vi "ProvaRobot.vi"() -> ()   [LabVIEW 2017]
uses:
  Sub VIs/Utilities/Start Boolean.ctl
  <vilib>/Platform/TimedLoop/XDataNode/timing_clust.ctl
  <vilib>/Platform/TimedLoop/XDataNode/nitl_modes.ctl
  <vilib>/Platform/TimedLoop/XDataNode/wakeup.ctl
  <vilib>/rvi/eio/common/nirviEmuTemplateMethod_errors.vi
  <vilib>/rvi/Emulation/niFpgaCriticalErrorInLSC.vi
  <vilib>/rvi/Emulation/niFpgaGetClockAttributes.vi
  <vilib>/rvi/Emulation/niFpgaEmulationReportErrorSimple.vi
  <vilib>/rvi/Emulation/niFpgaSctlEmulationGetInTimedLoop.vi
  <vilib>/rvi/eio/common/nirviEmuReportErrorAndStop.vi
  <vilib>/rvi/DataTransferAndStorage/Container/Common/niFpgaContainerSetEmuInfo.vi
  <vilib>/rvi/DataTransferAndStorage/Container/Common/niFpgaContainerGetUniqueNameForEmu.vi
  <vilib>/rvi/Emulation/niFpgaProcessEmulError.vi
  <vilib>/rvi/FIFO/Fifo_Resource/nirvififoEmulationDetermineInputValidOut.vi
  <vilib>/rvi/errors/nirviReportUnexpectedCaseInternalError.vi
  <vilib>/rvi/errors/nirviReportUnexpectedCaseInternalError (U32).vi
  <vilib>/rvi/occurrence/nirviWaitOnOccurrenceBase.vi
  <vilib>/rvi/FIFO/Fifo_Resource/nirvififoEmulationReleaseLock.vi
  <vilib>/rvi/FIFO/Fifo_Resource/nirvififoEmulationObtainLock.vi
  <vilib>/rvi/FIFO/Fifo_Resource/nirvififoEmulationCreateLock.vi
  <vilib>/rvi/FIFO/Fifo_Resource/nirvififoEmulationSetSize.vi
  <vilib>/rvi/FIFO/Fifo_Resource/nirviFifoEmulationQueueMgr.vi
  <instcachedir>/0/nirviFifoEmulationQueueMgr_E5CAEC123FF24DC58D834DCA3CDAA9B5.lvgen/nirviFifoEmulationQueueMgr_E5CAEC123FF24DC58D834DCA3CDAA9B5_000.vi
  <vilib>/rvi/errors/niFpgaSetErrorForExecOnDevCompSimple.vi
  <vilib>/rvi/Emulation/niFpgaEmulationIsFPGAContextNoSignature.vi
  <vilib>/Utility/error.llb/Clear Errors.vi
  <vilib>/Platform/TimedLoop/XDataNode/XDataNode.xnode
  <vilib>/eio/EIOMethodNode/EIOMethodNode.xnode
  <vilib>/eio/EIONode/EIONode.xnode
  <vilib>/rvi/LocalResourceManager/LocalResourceManager.xnode
  <vilib>/rvi/DataTransferAndStorage/Container/XNode/niFpgaContainer.xnode
  <vilib>/rvi/FIFO/Fifo_Resource/nirvififoEmulationWrite.vi
  <vilib>/rvi/FIFO/Fifo_Resource/nirvififoEmulationRead.vi
  <vilib>/Platform/TimedLoop/XDataNode/XDNodeRunTimeDep.lvlib
panel:
  in  "enable aux":bool
  in  "Numeric":u8
  in  "invertiM4":bool=TRUE
  in  "InvertiM3":bool=TRUE
  in  "InvertiM2":bool=TRUE
  in  "InvertiM1":bool=TRUE
  in  "DIO.C_0:7_write 2":u8 format="%08b"
  in  "ENB_AB 2":bool
  in  "ENB_AB":bool
  in  "DO.LED3:0":u8 format="%04b"
  out "DI.BTN":u8 format="%08b"
  in  "IRQ.DI_BTN.ENA":bool
  in  "IRQ.DI_BTN.RISE":bool
  in  "IRQ.DI_BTN.FALL":bool
  in  "IRQ.DI_BTN.CNT":u32
  in  "IRQ.DI_BTN.NO":u8
  out "AI.A_0.VAL":u16
  out "AI.A_1.VAL":u16
  out "AI.A_2.VAL":u16
  out "AI.A_3.VAL":u16
  out "AI.B_0.VAL":u16
  out "AI.B_1.VAL":u16
  out "AI.B_2.VAL":u16
  out "AI.B_3.VAL":u16
  out "AI.AudioIn_L.VAL":u16
  out "AI.AudioIn_R.VAL":u16
  out "AI.C_1.VAL":u16
  out "AI.C_0.VAL":u16
  in  "IRQ.AI_A_3:0.CNFG":u8 format="%.0b"
  in  "IRQ.AI_A_0.THRESHOLD":u16
  in  "IRQ.AI_A_1.THRESHOLD":u16
  in  "IRQ.AI_A_0.NO":u8
  in  "IRQ.AI_A_1.NO":u8
  in  "IRQ.AI_A_1.HYSTERESIS":u16=17
  in  "IRQ.AI_A_0.HYSTERESIS":u16=17
  in  "IRQ.TIMER.SETTIME":T1
  in  "IRQ.TIMER.WRITE":u32
  out "IRQ.TIMER.READ":u32
  out "SYS.RDY":bool
  out "SYS.AI.RDY":bool
  out "ACC.Z.VAL":u16
  out "SYS.ACC.RDY":bool
  out "ACC.Y.VAL":u16
  out "ACC.X.VAL":u16
  in  "StartShiftReg":bool
  in  "enable cannon":bool
  in  "SYS.SELECTA":u8 format="%08b"
  in  "DIO.A_15:8.OUT":u8 format="%08b"
  in  "DIO.A_15:8.DIR":u8 format="%08b"
  in  "I2C.A.DATO":u8
  out "I2C.A.DATI":u8
  in  "I2C.A.ADDR":u8 format="%08b"
  in  "I2C.A.CNTR":u8=213
  in  "I2C.A.CNTL":u8 format="%08b"
  out "I2C.A.STAT":u8 format="%08b"
  in  "I2C.A.CNFG":u8=1 format="%08b"
  in  "I2C.A.GO":T1
  in  "PWM period motor 4":u16=4000
  in  "Duty cycle motor 4":i16
  in  "PWM period motor 3":u16=4000
  in  "Duty cycle motor 3":i16
  out "deltaT motor 4":i32
  in  "Clear Overflow? 7":bool
  out "StatusEnc 7":u8
  out "Count encoder motor 4":u32
  in  "Reset encoder motor 4":bool
  out "deltaT motor 3":i32
  in  "Clear Overflow? 6":bool
  out "StatusEnc 6":u8
  out "Count encoder motor 3":u32
  in  "Reset encoder motor 3":bool
  in  "Reset encoder motor 1":bool
  out "Count encoder motor 1":u32
  out "StatusEnc 5":u8
  in  "Clear Overflow? 5":bool
  out "deltaT motor 1":i32
  in  "Reset encoder motor 2":bool
  out "Count encoder motor 2":u32
  out "StatusEnc 4":u8
  in  "Clear Overflow? 4":bool
  out "deltaT motor 2":i32
  in  "Duty cycle motor 1":i16
  in  "PWM period motor 1":u16=4000
  in  "Duty cycle motor 2":i16
  in  "PWM period motor 2":u16=4000
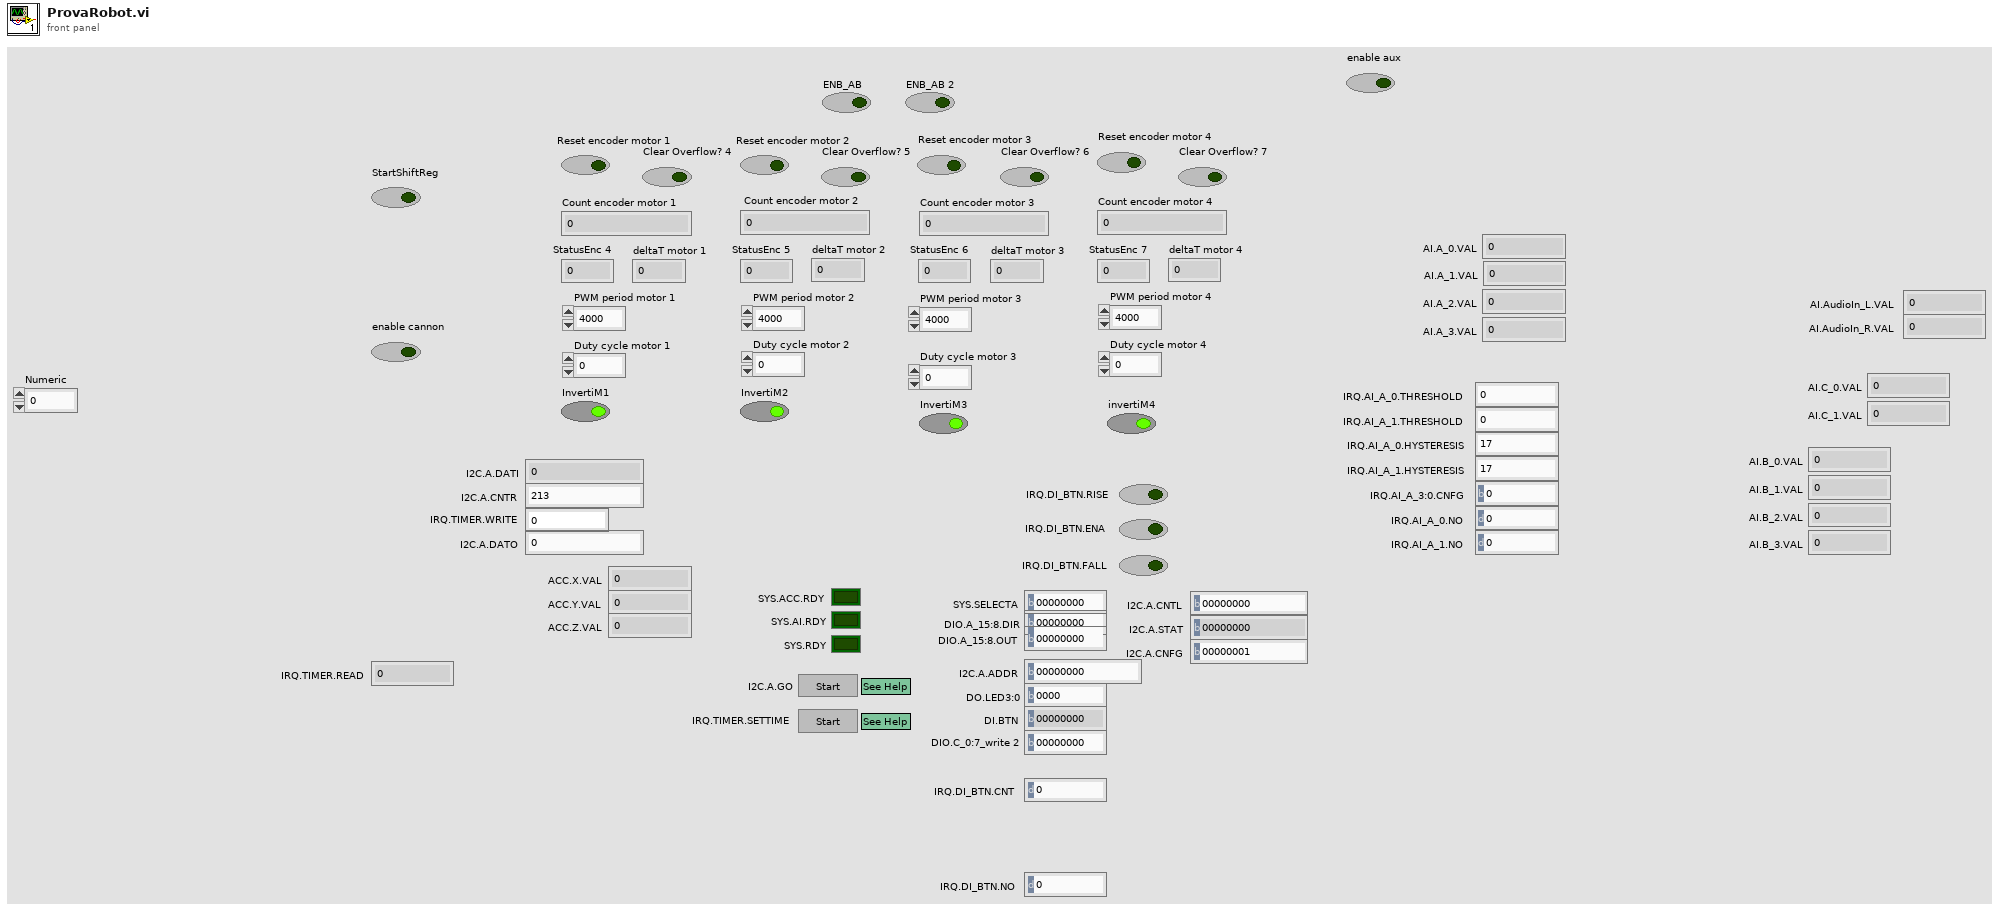
[diagram p1: front panel]
types:
  T1 = typedef "Start Boolean.ctl" = bool
  T2 = typedef "XDNodeRunTimeDep.lvlib/timing_clust.ctl" = cluster{"Expected End [f-1]":u64, "Actual End [f-1]":u64, "Finished Late? [f-1]":bool, "Expected End [i-1]":u64, "Actual End [i-1]":u64, "Finished Late? [i-1]":bool, "Expected Start [i]":u64, "Actual Start [i]":u64, "Expected Start [f]":u64, "Actual Start [f]":u64, "Source Name":string, "Structure Name":string, "Period":i64, "Deadline":i64, "Offset":i64, "Start":i64, "Priority":i32, "Timeout":i32, "Mode":T3, "Wakeup Reason":T4, "Error":errorcluster, "Source Type":string, "Secondary Source Type":string, "Global End Time":u64, "Global Start Time":u64, "Frame Duration":u64, "Iteration Duration":u64, "Assigned CPU":i32, "I/O Scan Engine Mode":u32}
  T3 = typedef "XDNodeRunTimeDep.lvlib/nitl_modes.ctl" = enum32{"No Change", "Process missed periods, maintain original phase", "Discard missed periods, maintain original phase", "Process missed periods, ignore original phase", "Discard missed periods, ignore original phase"}
  T4 = typedef "XDNodeRunTimeDep.lvlib/wakeup.ctl" = enum32{"Normal", "Aborted", "Asynchronous wakeup", "Timing source error", "Timed loop error", "Timeout"}
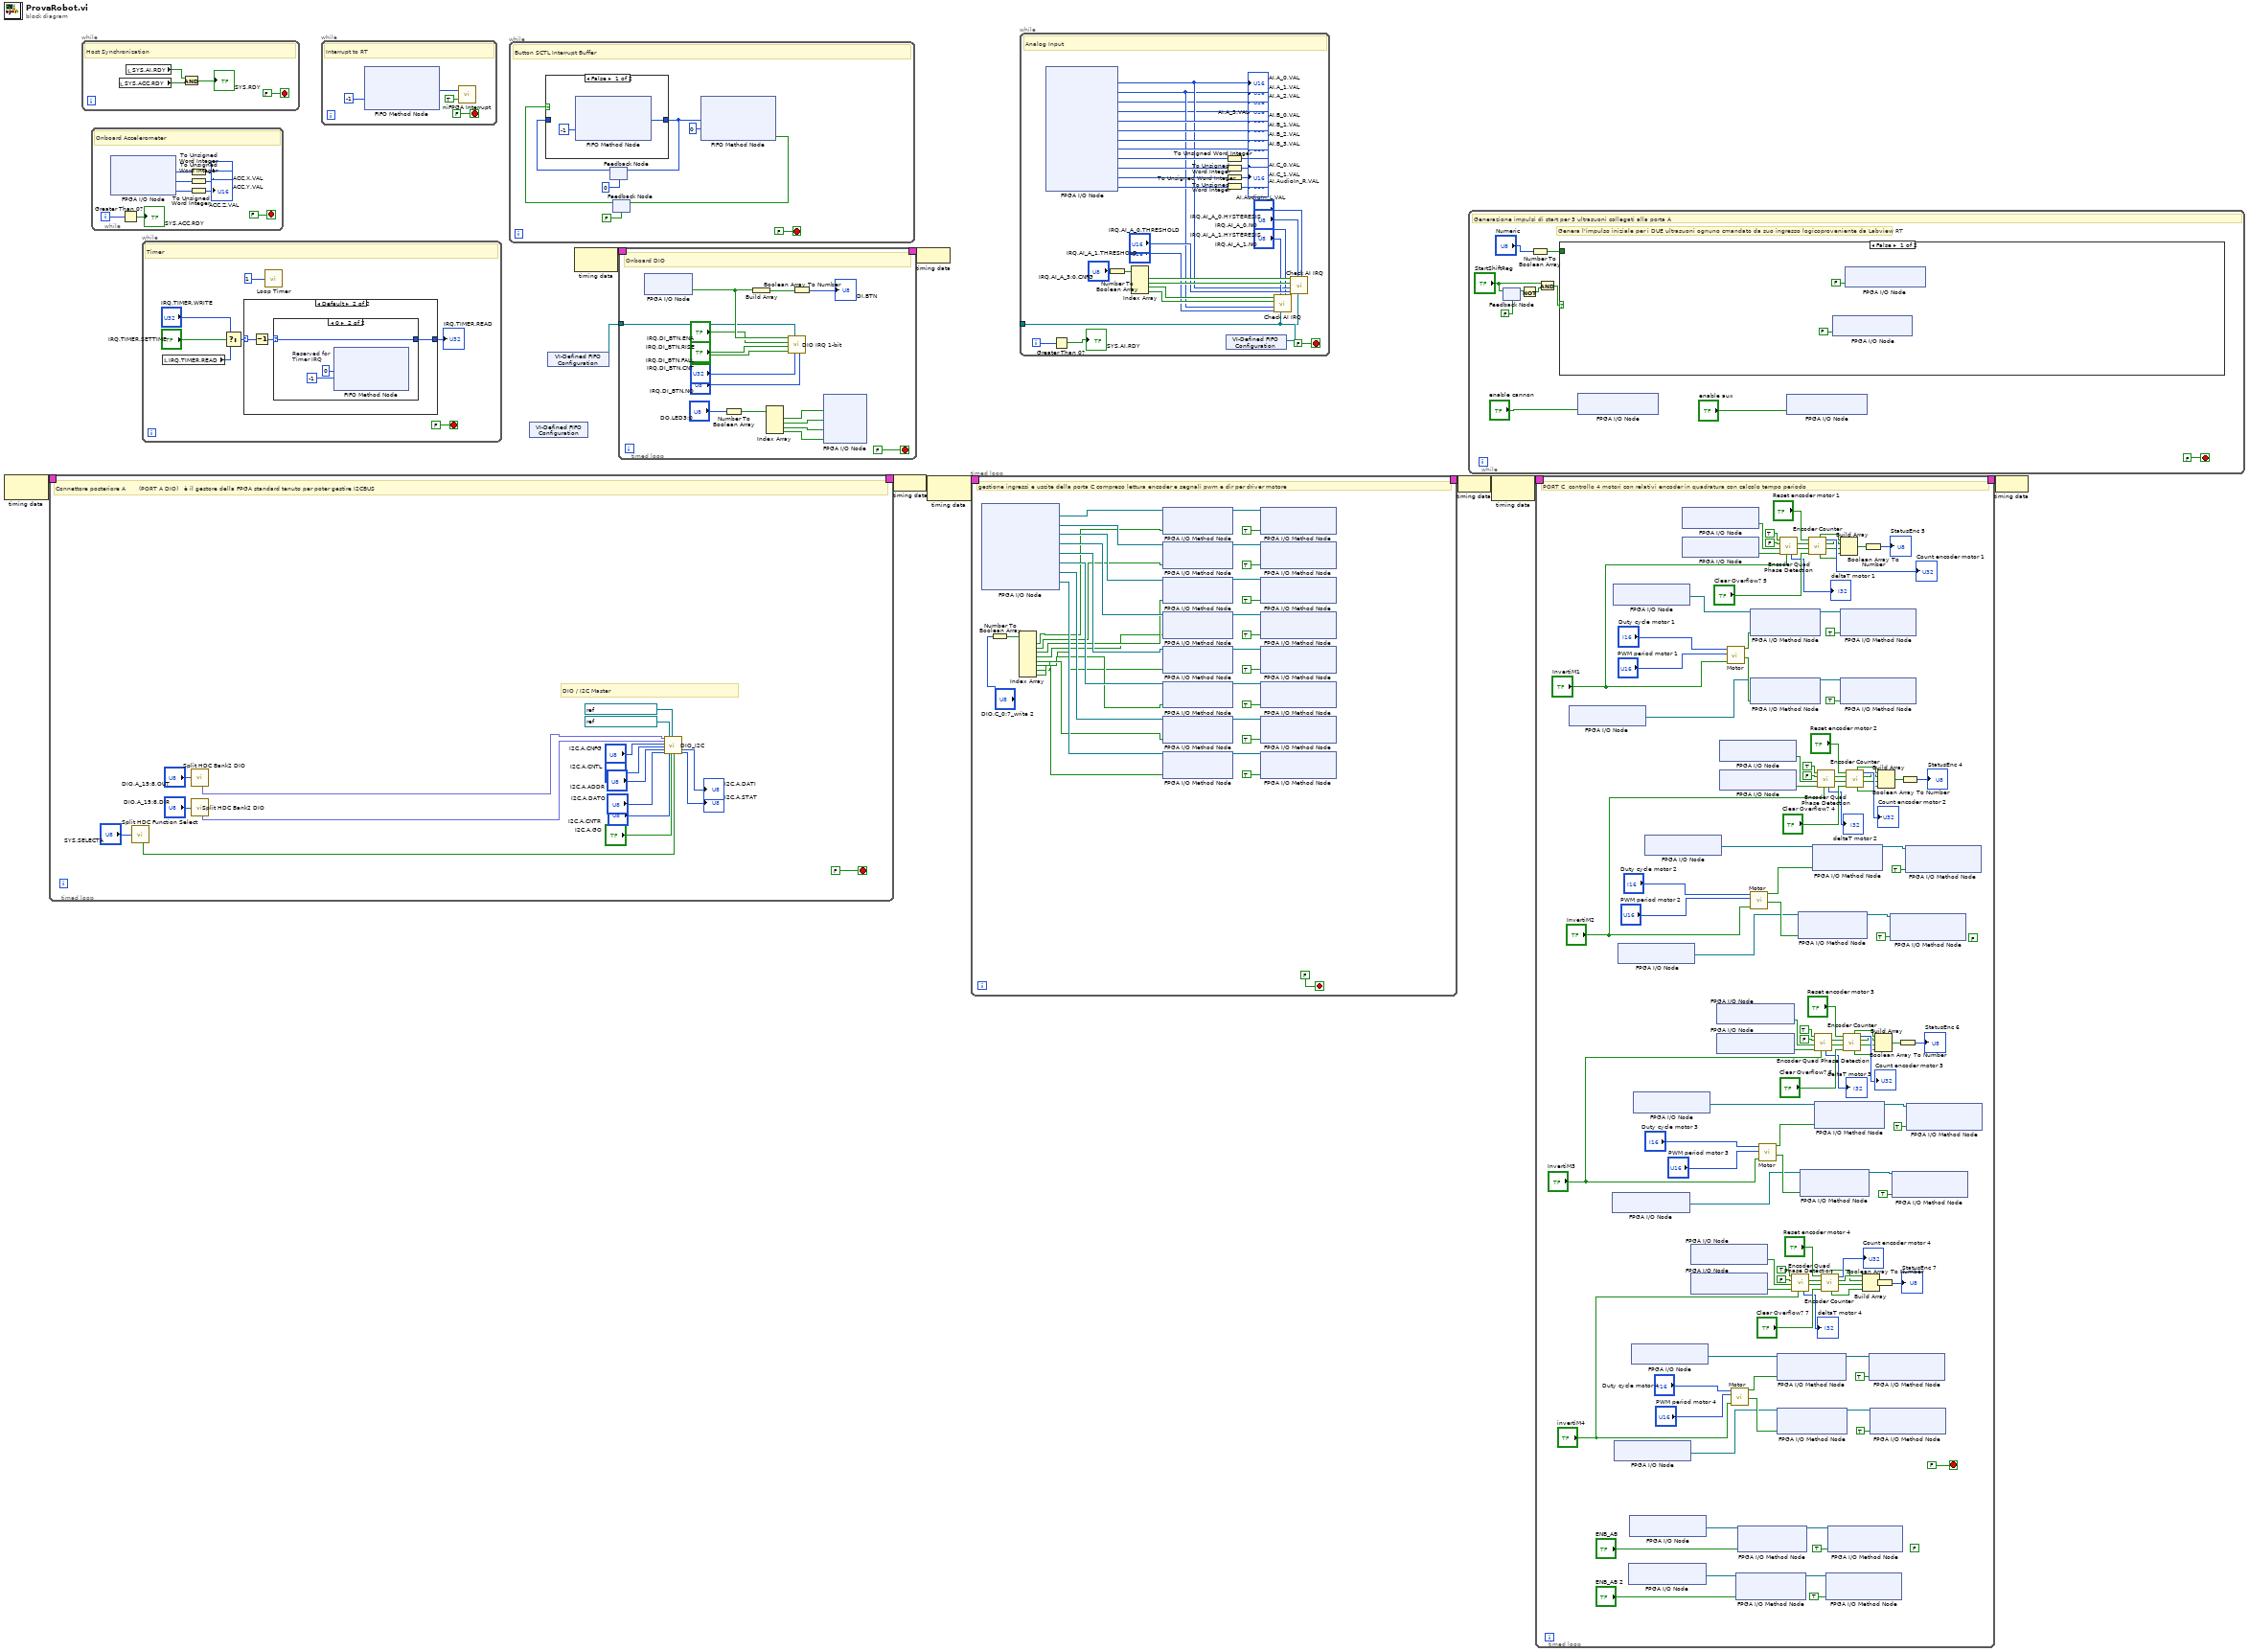
[diagram p0: block diagram]
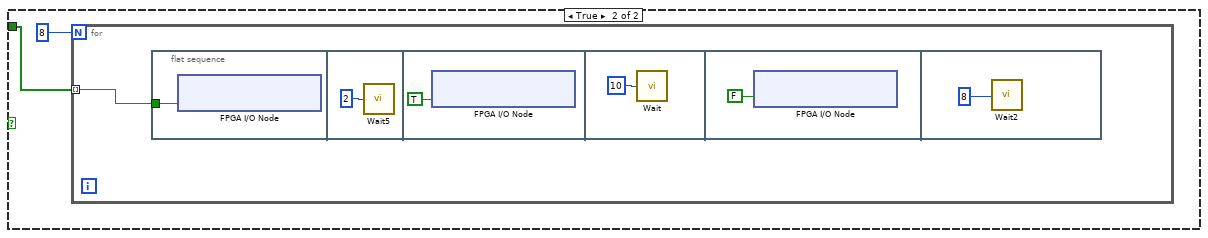
[diagram p5: hidden frame]
diagram:
  n1 = node-c288() -> (w6:T2)  [unwired: 1 in]
  n2 = timed-loop {
    timing: w6 -> [_]
    timing-out: [_] -> w5
    stop <- FALSE stop-if-true
    # "DIO / I2C Master"
    # "Connettore posteriore A       (PORT A DIO)   è il gestore della FPGA standard tenuto per poter gestire I2CBUS"
    n3 = call "Split HDC Function Select.vi"("IN 7:0"="SYS.SELECTA") -> ("OUT 7"=w12:bool)  [unwired: 5 out]
    n4 = call "Split HDC Bank2 DIO.vi"("IN 7:0"="DIO.A_15:8.OUT") -> ("OUT 7:6"=w15:fxp<+,2,2>)  [unwired: 2 in, 5 out]
    n5 = call "Split HDC Bank2 DIO.vi"("IN 7:0"="DIO.A_15:8.DIR") -> ("OUT 7:6"=w14:fxp<+,2,2>)  [unwired: 2 in, 5 out]
    n6 = call "DIO_I2C.vi"("DIO.1:0.OUT"=w15, "DIO.1:0.DIR"=w14, "I2C.CNFG"="I2C.A.CNFG", "I2C.CNTL"="I2C.A.CNTL", "I2C.ADDR"="I2C.A.ADDR", "I2C.DATO"="I2C.A.DATO", "DIO.1/I2C.SDA"=refnum<k21> "ConnectorA/DIO15" ("DIO.1/I2C.SCL"), "I2C.CNTR"="I2C.A.CNTR", "DIO.0/I2C.SCL"=refnum<k21> "ConnectorA/DIO14" ("DIO.0/I2C.SDA"), "Execute?"="I2C.A.GO", "SELECT"=w12) -> ("I2C.DATI"=→"I2C.A.DATI":u8, "I2C.STAT"=→"I2C.A.STAT":u8)  [unwired: 6 in, 1 out]
  }
  n7 = while {
    stop <- FALSE stop-if-true
    # "Host Synchronization"
    n8 = local read "SYS.ACC.RDY"() -> (w31:bool)
    n9 = local read "SYS.AI.RDY"() -> (w33:bool)
    n10 = Compound Arithmetic op=AND(w33, w31) -> (→"SYS.RDY":bool)
  }
  n11 = while {
    i -> [w38]
    stop <- FALSE stop-if-true
    # "Onboard Accelerometer"
    n12 = xnode "FPGA I/O Node"() -> ("AccelerationX"=w41:i16, "AccelerationY"=w40:i16, "AccelerationZ"=w39:i16)  [unwired: 3 in, 3 out]
    n13 = Greater Than 0?(x=w38) -> (x > 0?=→"SYS.ACC.RDY":bool)
    n14 = To Unsigned Word Integer(number=w41) -> (unsigned 16bit integer=→"ACC.X.VAL":u16)
    n15 = To Unsigned Word Integer(number=w40) -> (unsigned 16bit integer=→"ACC.Y.VAL":u16)
    n16 = To Unsigned Word Integer(number=w39) -> (unsigned 16bit integer=→"ACC.Z.VAL":u16)
  }
  n17 = while {
    stop <- FALSE stop-if-true
    # "Timer"
    n18 = local read "IRQ.TIMER.READ"() -> (w46:u32)
    n19 = Select(t="IRQ.TIMER.WRITE", s="IRQ.TIMER.SETTIME", f=w46) -> (s? t:f=w44:u32)
    n20 = case shown="Default" w44 {
      selector: w44 -> [w50 w53]
      tunnel: [w50 w51] -> w43
      frame 0 {
      }
      frame Default {
        n21 = Decrement(x=w53) -> (x-1=w52:u32)
        n22 = case shown="0" w52 {
          selector: w52 -> [w54 w57]
          tunnel: [w54 w57] -> w51
          frame Default {
          }
          frame 0 {
            w56 = u8 0  # Reserved for Timer IRQ
            n23 = xnode ("FIFO Method Node")("Element"=w56, "Timeout"=-1) -> ()  [unwired: 1 in, 2 out]
          }
        }
      }
    }
    "IRQ.TIMER.READ" <- w43
    n24 = call "Loop Timer"("Count(uSec)"=u8 1 ("Count(mSec)")) -> ()  [unwired: 1 out]
  }
  n25 = while {
    stop <- FALSE stop-if-true
    # "Interrupt to RT"
    n26 = xnode ("FIFO Method Node")("Timeout"=-1) -> ("Element"=w60:u8)  [unwired: 1 in, 2 out]
    n27 = call <vilib>:"niFPGA Interrupt.vi"("Wait Until Cleared (F)"=TRUE, "IRQ Number (0)"=w60) -> ()  [unwired: 1 in]
  }
  n28 = while {
    stop <- FALSE stop-if-true
    # "Button SCTL Interrupt Buffer"
    n29 = feedback #1(u8 0 ("Element")) -> (w64:u8)
    n30 = feedback #2(FALSE ("Timed Out?")) -> (w68:bool)
    n31 = case shown="False" w68 {
      tunnel: [w70 w72] -> w65
      tunnel: w64 -> [_ w72]
      frame False {
        n32 = xnode ("FIFO Method Node")("Timeout"=-1) -> ("Element"=w70:u8)  [unwired: 1 in, 2 out]
      }
      frame True {
      }
    }
    n33 = feedback-in #1(w65) -> ()
    n34 = xnode ("FIFO Method Node")("Element"=w65, "Timeout"=0) -> ("Timed Out?"=w66:bool)  [unwired: 1 in, 1 out]
    n35 = feedback-in #2(w66) -> ()
  }
  n36 = xnode "VI-Defined FIFO Configuration"() -> ()  [unwired: 1 out]
  n37 = xnode "VI-Defined FIFO Configuration"() -> ("FIFO Out"=w1:refnum<k21>)
  n38 = node-c288() -> (w3:T2)  [unwired: 1 in]
  n39 = timed-loop {
    timing: w3 -> [_]
    timing-out: [_] -> w2
    tunnel: w1 -> [w76]
    stop <- FALSE stop-if-true
    # "Onboard DIO"
    n40 = xnode "FPGA I/O Node"() -> ("Button0"=w80:bool)  [unwired: 1 in, 1 out]
    n41 = Number To Boolean Array(number="DO.LED3:0") -> (Boolean array=w85:bool[])
    n42 = Build Array(w80) -> (w88:bool[])
    n43 = Index Array(array=w85) -> (element #1=w84:bool, element #2=w83:bool, element #3=w82:bool, element #4=w81:bool)  [unwired: 4 in]
    n44 = call "DIO IRQ 1-bit.vi"("IRQ.NO"="IRQ.DI_BTN.NO", "IRQ.CNT"="IRQ.DI_BTN.CNT", "FIFO in"=w76, "IRQ.FALL"="IRQ.DI_BTN.FALL", "IRQ.RISE"="IRQ.DI_BTN.RISE", "IRQ.ENA"="IRQ.DI_BTN.ENA", "DIO"=w80) -> ()  [unwired: 5 in]
    n45 = Boolean Array To Number(Boolean array=w88) -> (number=→"DI.BTN":u8)
    n46 = xnode "FPGA I/O Node"("LED0"=w84, "LED1"=w83, "LED2"=w82, "LED3"=w81) -> ()  [unwired: 4 in, 4 out]
  }
  n47 = node-c288(w5) -> ()
  n48 = node-c288(w2) -> ()
  n49 = node-c288() -> (w10:T2)  [unwired: 1 in]
  n50 = timed-loop {
    timing: w10 -> [_]
    timing-out: [_] -> w9
    stop <- FALSE stop-if-true
    # "gestione ingressi e uscite della porta C compreso lettura encoder e segnali pwm e dir per driver motore"
    n51 = xnode "FPGA I/O Node"() -> ("FPGA I/O Out"=w124:refnum<k21>, "FPGA I/O Out"=w111:refnum<k21>, "FPGA I/O Out"=w110:refnum<k21>, "FPGA I/O Out"=w105:refnum<k21>, "FPGA I/O Out"=w104:refnum<k21>, "FPGA I/O Out"=w103:refnum<k21>, "FPGA I/O Out"=w102:refnum<k21>, "FPGA I/O Out"=w101:refnum<k21>)  [unwired: 8 in, 8 out]
    n52 = Number To Boolean Array(number="DIO.C_0:7_write 2") -> (Boolean array=w100:bool[])
    n53 = Index Array(array=w100) -> (element #1=w98:bool, element #2=w97:bool, element #3=w96:bool, element #4=w95:bool, element #5=w91:bool, element #6=w92:bool, element #7=w93:bool, element #8=w94:bool)  [unwired: 8 in]
    n54 = xnode "FPGA I/O Method Node"("FPGA I/O In"=w124, "Data"=w98) -> ("FPGA I/O Out"=w123:refnum<k21>)
    n55 = xnode "FPGA I/O Method Node"("FPGA I/O In"=w111, "Data"=w97) -> ("FPGA I/O Out"=w121:refnum<k21>)
    n56 = xnode "FPGA I/O Method Node"("FPGA I/O In"=w110, "Data"=w96) -> ("FPGA I/O Out"=w119:refnum<k21>)
    n57 = xnode "FPGA I/O Method Node"("FPGA I/O In"=w105, "Data"=w95) -> ("FPGA I/O Out"=w117:refnum<k21>)
    n58 = xnode "FPGA I/O Method Node"("FPGA I/O In"=w104, "Data"=w91) -> ("FPGA I/O Out"=w115:refnum<k21>)
    n59 = xnode "FPGA I/O Method Node"("FPGA I/O In"=w103, "Data"=w92) -> ("FPGA I/O Out"=w113:refnum<k21>)
    n60 = xnode "FPGA I/O Method Node"("FPGA I/O In"=w102, "Data"=w93) -> ("FPGA I/O Out"=w109:refnum<k21>)
    n61 = xnode "FPGA I/O Method Node"("FPGA I/O In"=w101, "Data"=w94) -> ("FPGA I/O Out"=w107:refnum<k21>)
    n62 = xnode "FPGA I/O Method Node"("FPGA I/O In"=w123, "Enable"=TRUE) -> ()  [unwired: 1 out]
    n63 = xnode "FPGA I/O Method Node"("FPGA I/O In"=w121, "Enable"=TRUE) -> ()  [unwired: 1 out]
    n64 = xnode "FPGA I/O Method Node"("FPGA I/O In"=w119, "Enable"=TRUE) -> ()  [unwired: 1 out]
    n65 = xnode "FPGA I/O Method Node"("FPGA I/O In"=w117, "Enable"=TRUE) -> ()  [unwired: 1 out]
    n66 = xnode "FPGA I/O Method Node"("FPGA I/O In"=w115, "Enable"=TRUE) -> ()  [unwired: 1 out]
    n67 = xnode "FPGA I/O Method Node"("FPGA I/O In"=w113, "Enable"=TRUE) -> ()  [unwired: 1 out]
    n68 = xnode "FPGA I/O Method Node"("FPGA I/O In"=w109, "Enable"=TRUE) -> ()  [unwired: 1 out]
    n69 = xnode "FPGA I/O Method Node"("FPGA I/O In"=w107, "Enable"=TRUE) -> ()  [unwired: 1 out]
  }
  n70 = xnode "VI-Defined FIFO Configuration"() -> ("FIFO Out"=w4:refnum<k21>)
  n71 = while {
    tunnel: w4 -> [w130]
    i -> [w156]
    stop <- FALSE stop-if-true
    # "Analog Input"
    n72 = xnode "FPGA I/O Node"() -> ("ConnectorA/AI0"=w135:u16, "ConnectorA/AI1"=w134:u16, "ConnectorA/AI2"=→"AI.A_2.VAL":u16, "ConnectorA/AI3"=→"AI.A_3.VAL":u16, "ConnectorB/AI0"=→"AI.B_0.VAL":u16, "ConnectorB/AI1"=→"AI.B_1.VAL":u16, "ConnectorB/AI2"=→"AI.B_2.VAL":u16, "ConnectorB/AI3"=→"AI.B_3.VAL":u16, "ConnectorC/AI0"=w151:i16, "ConnectorC/AI1"=w150:i16, "AudioIn/Left"=w149:i16, "AudioIn/Right"=w148:i16)  [unwired: 12 in, 12 out]
    "AI.A_0.VAL" <- w135
    "AI.A_1.VAL" <- w134
    n73 = Greater Than 0?(x=w156) -> (x > 0?=→"SYS.AI.RDY":bool)
    n74 = Number To Boolean Array(number="IRQ.AI_A_3:0.CNFG") -> (Boolean array=w145:bool[])
    n75 = Index Array(array=w145) -> (element #1=w143:bool, element #2=w142:bool, element #3=w140:bool, element #4=w139:bool)  [unwired: 4 in]
    n76 = To Unsigned Word Integer(number=w151) -> (unsigned 16bit integer=→"AI.C_0.VAL":u16)
    n77 = To Unsigned Word Integer(number=w150) -> (unsigned 16bit integer=→"AI.C_1.VAL":u16)
    n78 = To Unsigned Word Integer(number=w149) -> (unsigned 16bit integer=→"AI.AudioIn_L.VAL":u16)
    n79 = To Unsigned Word Integer(number=w148) -> (unsigned 16bit integer=→"AI.AudioIn_R.VAL":u16)
    n80 = call "Check AI IRQ.vi"("Hysteresis"="IRQ.AI_A_1.HYSTERESIS", "FIFO In"=w130, "IRQ Number"="IRQ.AI_A_1.NO", "Threshold"="IRQ.AI_A_1.THRESHOLD", "Analog Value"=w134, "Rising Edge?"=w139, "Enable Interrupt?"=w140) -> ()  [unwired: 5 in]
    n81 = call "Check AI IRQ.vi"("Hysteresis"="IRQ.AI_A_0.HYSTERESIS", "FIFO In"=w130, "IRQ Number"="IRQ.AI_A_0.NO", "Threshold"="IRQ.AI_A_0.THRESHOLD", "Analog Value"=w135, "Rising Edge?"=w142, "Enable Interrupt?"=w143) -> ()  [unwired: 5 in]
  }
  n82 = node-c288(w9) -> ()
  n83 = while {
    stop <- FALSE stop-if-true
    # "Genera l'impulso iniziale per i DUE ultrasuoni ognuno cmandato da suo ingresso logicoproveniente da Labview RT"
    # "Generazione impulsi di start per 3 ultrasuoni collegati alla porta A"
    n84 = feedback-in #3("StartShiftReg") -> ()
    n85 = feedback #3(FALSE ("StartShiftReg")) -> (w167:bool)
    n86 = Not(x=w167) -> (.not. x?=w168:bool)
    n87 = Number To Boolean Array(number="Numeric") -> (Boolean array=w162:bool[])
    n88 = And(x="StartShiftReg", y=w168) -> (x .and. y?=w164:bool)
    n89 = case shown="False" w164 {
      tunnel: w162 -> [_ w173]
      frame False {
        n90 = xnode "FPGA I/O Node"("ConnectorB/DIO10"=FALSE ("ConnectorB/DIO13")) -> ()  [unwired: 1 in, 1 out]
        n91 = xnode "FPGA I/O Node"("ConnectorB/DIO13"=FALSE) -> ()  [unwired: 1 in, 1 out]
      }
      frame True {
        n92 = for {
          N: 8 -> [_]
          tunnel: w173 -> [w174] mode=indexing
          n93 = flat-sequence {
            tunnel: w174 -> [w175]
            frame #0 {
              n94 = xnode "FPGA I/O Node"("ConnectorB/DIO10"=w175) -> ()  [unwired: 1 in, 1 out]
            }
            frame #1 {
              n95 = call "Wait5"("Count(uSec)"=u32 2) -> ()  [unwired: 1 out]
            }
            frame #2 {
              n96 = xnode "FPGA I/O Node"("ConnectorB/DIO13"=TRUE) -> ()  [unwired: 1 in, 1 out]
            }
            frame #3 {
              n97 = call "Wait"("Count(uSec)"=u32 10) -> ()  [unwired: 1 out]
            }
            frame #4 {
              n98 = xnode "FPGA I/O Node"("ConnectorB/DIO13"=FALSE ("ConnectorC/DIO6")) -> ()  [unwired: 1 in, 1 out]
            }
            frame #5 {
              n99 = call "Wait2"("Count(mSec)"=u32 8 ("Count(uSec)")) -> ()  [unwired: 1 out]
            }
          }
        }
      }
    }
    n100 = xnode "FPGA I/O Node"("ConnectorB/DIO12"="enable cannon") -> ()  [unwired: 1 in, 1 out]
    n101 = xnode "FPGA I/O Node"("ConnectorB/DIO11"="enable aux") -> ()  [unwired: 1 in, 1 out]
  }
  n102 = node-c288() -> (w8:T2)  [unwired: 1 in]
  n103 = timed-loop "Timed Loop" {
    timing: w8 -> [_]
    timing-out: [_] -> w7
    stop <- FALSE stop-if-true
    (unwired) FALSE
    (unwired) FALSE
    # "PORT C  controllo 4 motori con relativi encoder in quadratura con calcolo tempo periodo"
    n104 = xnode "FPGA I/O Node"() -> ("FPGA I/O Out"=w185:refnum<k21>)  [unwired: 1 in, 1 out]
    n105 = xnode "FPGA I/O Node"() -> ("FPGA I/O Out"=w191:refnum<k21>)  [unwired: 1 in, 1 out]
    n106 = xnode "FPGA I/O Node"() -> ("FPGA I/O Out"=w186:refnum<k21>)  [unwired: 1 in, 1 out]
    n107 = xnode "FPGA I/O Node"() -> ("FPGA I/O Out"=w189:refnum<k21>)  [unwired: 1 in, 1 out]
    n108 = xnode "FPGA I/O Node"() -> ("FPGA I/O Out"=w187:refnum<k21>)  [unwired: 1 in, 1 out]
    n109 = xnode "FPGA I/O Node"() -> ("FPGA I/O Out"=w194:refnum<k21>)  [unwired: 1 in, 1 out]
    n110 = xnode "FPGA I/O Node"() -> ("FPGA I/O Out"=w198:refnum<k21>)  [unwired: 1 in, 1 out]
    n111 = xnode "FPGA I/O Node"() -> ("FPGA I/O Out"=w190:refnum<k21>)  [unwired: 1 in, 1 out]
    n112 = xnode "FPGA I/O Node"() -> ("FPGA I/O Out"=w192:refnum<k21>)  [unwired: 1 in, 1 out]
    n113 = xnode "FPGA I/O Node"() -> ("FPGA I/O Out"=w188:refnum<k21>)  [unwired: 1 in, 1 out]
    n114 = xnode "FPGA I/O Node"() -> ("ConnectorB/DIO3"=w296:bool)  [unwired: 1 in, 1 out]
    n115 = xnode "FPGA I/O Node"() -> ("ConnectorB/DIO2"=w295:bool)  [unwired: 1 in, 1 out]
    n116 = xnode "FPGA I/O Node"() -> ("ConnectorA/DIO8"=w232:bool)  [unwired: 1 in, 1 out]
    n117 = xnode "FPGA I/O Node"() -> ("ConnectorA/DIO9"=w231:bool)  [unwired: 1 in, 1 out]
    n118 = xnode "FPGA I/O Node"() -> ("ConnectorA/DIO2"=w248:bool)  [unwired: 1 in, 1 out]
    n119 = xnode "FPGA I/O Node"() -> ("ConnectorA/DIO3"=w247:bool)  [unwired: 1 in, 1 out]
    n120 = xnode "FPGA I/O Node"() -> ("ConnectorB/DIO9"=w280:bool)  [unwired: 1 in, 1 out]
    n121 = xnode "FPGA I/O Node"() -> ("ConnectorB/DIO8"=w279:bool)  [unwired: 1 in, 1 out]
    n122 = call "Motor.vi"("INVERTI"="InvertiM1", "Fine"="PWM period motor 1", "Change"="Duty cycle motor 1") -> ("OutB"=w261:bool, "outA"=w258:bool)  [unwired: 7 in]
    n123 = call "Motor.vi"("INVERTI"="invertiM4", "Fine"="PWM period motor 4", "Change"="Duty cycle motor 4") -> ("OutB"=w204:bool, "outA"=w209:bool)  [unwired: 7 in]
    n124 = xnode "FPGA I/O Method Node"("FPGA I/O In"=w194, "Data"="ENB_AB 2") -> ("FPGA I/O Out"=w196:refnum<k21>)
    n125 = xnode "FPGA I/O Method Node"("FPGA I/O In"=w198, "Data"="ENB_AB") -> ("FPGA I/O Out"=w200:refnum<k21>)
    n126 = xnode "FPGA I/O Method Node"("FPGA I/O In"=w186, "Data"=w258) -> ("FPGA I/O Out"=w264:refnum<k21>)
    n127 = xnode "FPGA I/O Method Node"("FPGA I/O In"=w185, "Data"=w261) -> ("FPGA I/O Out"=w263:refnum<k21>)
    n128 = call "Motor.vi"("INVERTI"="InvertiM2", "Fine"="PWM period motor 2", "Change"="Duty cycle motor 2") -> ("OutB"=w252:bool, "outA"=w257:bool)  [unwired: 7 in]
    n129 = call "Motor.vi"("INVERTI"="InvertiM3", "Fine"="PWM period motor 3", "Change"="Duty cycle motor 3") -> ("OutB"=w213:bool, "outA"=w210:bool)  [unwired: 7 in]
    n130 = xnode "FPGA I/O Method Node"("FPGA I/O In"=w190, "Data"=w209) -> ("FPGA I/O Out"=w208:refnum<k21>)
    n131 = xnode "FPGA I/O Method Node"("FPGA I/O In"=w189, "Data"=w204) -> ("FPGA I/O Out"=w206:refnum<k21>)
    n132 = call "Encoder Quad Phase Detection.vi"("direzione"="InvertiM1", "Phase B"=w295, "Phase A"=w296, "Clear Error?"=FALSE, "Enable?"=TRUE) -> ("Signal"=w291:bool, "Backward?"=w292:bool, "deltaT"=→"deltaT motor 1":i32)  [unwired: 3 in, 1 out]
    n133 = call "Encoder Quad Phase Detection.vi"("direzione"="invertiM4", "Phase B"=w231, "Phase A"=w232, "Clear Error?"=FALSE, "Enable?"=TRUE) -> ("Signal"=w227:bool, "Backward?"=w228:bool, "deltaT"=→"deltaT motor 4":i32)  [unwired: 3 in, 1 out]
    n134 = xnode "FPGA I/O Method Node"("FPGA I/O In"=w187, "Data"=w252) -> ("FPGA I/O Out"=w254:refnum<k21>)
    n135 = xnode "FPGA I/O Method Node"("FPGA I/O In"=w191, "Data"=w213) -> ("FPGA I/O Out"=w215:refnum<k21>)
    n136 = call "Encoder Counter.vi"("Clear Overflow?"="Clear Overflow? 5", "Signal"=w291, "Backward?"=w292, "Reset?"="Reset encoder motor 1") -> ("Crossed Halfway?"=w286:bool, "Wrapped around?"=w288:bool, "Count Value"=→"Count encoder motor 1":u32, "Crossed Halfway twice?"=w285:bool, "Wrapped around twice?"=w287:bool)  [unwired: 3 in]
    n137 = xnode "FPGA I/O Method Node"("FPGA I/O In"=w188, "Data"=w257) -> ("FPGA I/O Out"=w256:refnum<k21>)
    n138 = call "Encoder Quad Phase Detection.vi"("direzione"="InvertiM3", "Phase B"=w247, "Phase A"=w248, "Clear Error?"=FALSE, "Enable?"=TRUE) -> ("Signal"=w243:bool, "Backward?"=w244:bool, "deltaT"=→"deltaT motor 3":i32)  [unwired: 3 in, 1 out]
    n139 = xnode "FPGA I/O Method Node"("FPGA I/O In"=w192, "Data"=w210) -> ("FPGA I/O Out"=w216:refnum<k21>)
    n140 = call "Encoder Quad Phase Detection.vi"("direzione"="InvertiM2", "Phase B"=w279, "Phase A"=w280, "Clear Error?"=FALSE, "Enable?"=TRUE) -> ("Signal"=w275:bool, "Backward?"=w276:bool, "deltaT"=→"deltaT motor 2":i32)  [unwired: 3 in, 1 out]
    n141 = call "Encoder Counter.vi"("Clear Overflow?"="Clear Overflow? 7", "Signal"=w227, "Backward?"=w228, "Reset?"="Reset encoder motor 4") -> ("Crossed Halfway?"=w222:bool, "Wrapped around?"=w224:bool, "Count Value"=→"Count encoder motor 4":u32, "Crossed Halfway twice?"=w221:bool, "Wrapped around twice?"=w223:bool)  [unwired: 3 in]
    n142 = xnode "FPGA I/O Method Node"("FPGA I/O In"=w196, "Enable"=TRUE) -> ()  [unwired: 1 out]
    n143 = xnode "FPGA I/O Method Node"("FPGA I/O In"=w200, "Enable"=TRUE) -> ()  [unwired: 1 out]
    n144 = Build Array(w288, w287, w286, w285) -> (w284:bool[])
    n145 = xnode "FPGA I/O Method Node"("FPGA I/O In"=w264, "Enable"=TRUE) -> ()  [unwired: 1 out]
    n146 = xnode "FPGA I/O Method Node"("FPGA I/O In"=w263, "Enable"=TRUE) -> ()  [unwired: 1 out]
    n147 = call "Encoder Counter.vi"("Clear Overflow?"="Clear Overflow? 6", "Signal"=w243, "Backward?"=w244, "Reset?"="Reset encoder motor 3") -> ("Crossed Halfway?"=w238:bool, "Wrapped around?"=w240:bool, "Count Value"=→"Count encoder motor 3":u32, "Crossed Halfway twice?"=w237:bool, "Wrapped around twice?"=w239:bool)  [unwired: 3 in]
    n148 = call "Encoder Counter.vi"("Clear Overflow?"="Clear Overflow? 4", "Signal"=w275, "Backward?"=w276, "Reset?"="Reset encoder motor 2") -> ("Crossed Halfway?"=w270:bool, "Wrapped around?"=w272:bool, "Count Value"=→"Count encoder motor 2":u32, "Crossed Halfway twice?"=w269:bool, "Wrapped around twice?"=w271:bool)  [unwired: 3 in]
    n149 = Build Array(w224, w223, w222, w221) -> (w220:bool[])
    n150 = Boolean Array To Number(Boolean array=w284) -> (number=→"StatusEnc 5":u8)
    n151 = xnode "FPGA I/O Method Node"("FPGA I/O In"=w208, "Enable"=TRUE) -> ()  [unwired: 1 out]
    n152 = xnode "FPGA I/O Method Node"("FPGA I/O In"=w206, "Enable"=TRUE) -> ()  [unwired: 1 out]
    n153 = Build Array(w240, w239, w238, w237) -> (w236:bool[])
    n154 = Boolean Array To Number(Boolean array=w220) -> (number=→"StatusEnc 7":u8)
    n155 = Build Array(w272, w271, w270, w269) -> (w268:bool[])
    n156 = xnode "FPGA I/O Method Node"("FPGA I/O In"=w254, "Enable"=TRUE) -> ()  [unwired: 1 out]
    n157 = xnode "FPGA I/O Method Node"("FPGA I/O In"=w215, "Enable"=TRUE) -> ()  [unwired: 1 out]
    n158 = Boolean Array To Number(Boolean array=w236) -> (number=→"StatusEnc 6":u8)
    n159 = Boolean Array To Number(Boolean array=w268) -> (number=→"StatusEnc 4":u8)
    n160 = xnode "FPGA I/O Method Node"("FPGA I/O In"=w256, "Enable"=TRUE) -> ()  [unwired: 1 out]
    n161 = xnode "FPGA I/O Method Node"("FPGA I/O In"=w216, "Enable"=TRUE) -> ()  [unwired: 1 out]
  }
  n162 = node-c288(w7) -> ()
